vi "Untitled 25.vi"() -> ()   [LabVIEW 2019]
uses:
  examples/route_guide/route_guide_client/RPC Messages/routeguide_RouteSummary.ctl
  Generated_client/Generated_client.lvlib
  examples/route_guide/route_guide_client/route_guide_client.lvlib
panel:
  out "error out":errorcluster
  in  "error in":errorcluster
  in  "Longitude Loop":i32=4
  in  "Latitude Loop":i32=4
  in  "ms per iteration":u32=200
  out "Response Data":T1
  in  "Server Address":string="localhost:50051"
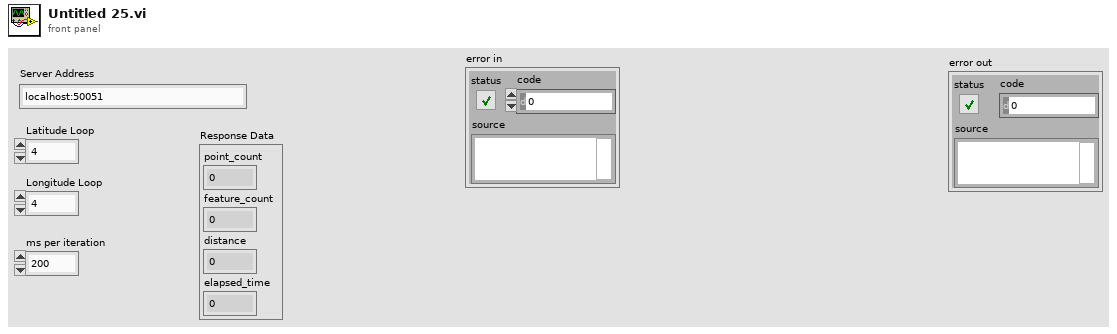
[diagram p1: front panel]
types:
  T1 = typedef "route_guide_client.lvlib/routeguide_RouteSummary.ctl" = cluster{"point_count":i32, "feature_count":i32, "distance":i32, "elapsed_time":i32}
  T2 = typedef "grpc-lvsupport-release.lvlib/grpcId.ctl" = u64
  T3 = typedef "Generated_client.lvlib/routeguide_RouteSummary.ctl" = cluster{"point_count":i32, "feature_count":i32, "distance":i32, "elapsed_time":i32}
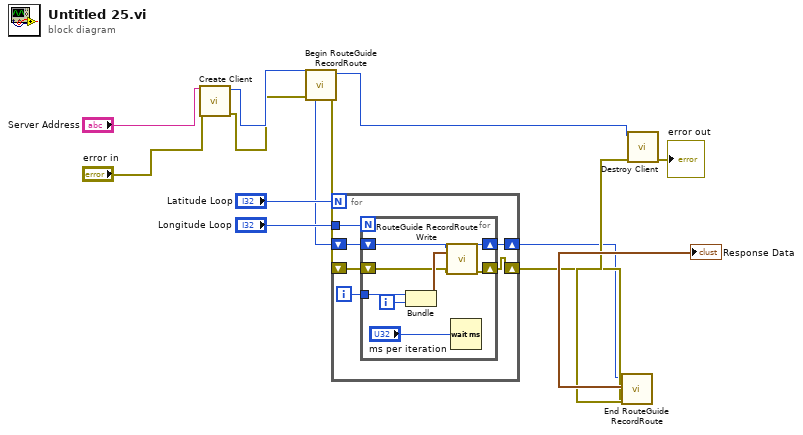
[diagram p0: block diagram]
diagram:
  n1 = call "Create Client.vi"("error in"="error in", "address"="Server Address") -> ("error out"=w5:errorcluster, "gRPC ID Out"=w9:T2)  [unwired: 8 in]
  n2 = call "Begin RouteGuide RecordRoute.vi"("error in"=w5, "gRPC ID"=w9) -> ("error out"=w6:errorcluster, "Call Id Out"=w7:T2, "gRPC ID out"=w8:T2)  [unwired: 7 in]
  n3 = for {
    N: "Latitude Loop" -> [_]
    shift-right: [w18] -> w1
    shift-left: w7 -> [w20]
    shift-right: [w15] -> w2
    shift-left: w6 -> [w19]
    tunnel: "Longitude Loop" -> [w16]
    i -> [w17]
    n4 = for {
      N: w16 -> [_]
      shift-right: [w22] -> w18
      shift-left: w20 -> [w25]
      shift-right: [w21] -> w15
      shift-left: w19 -> [w23]
      tunnel: w17 -> [w27]
      i -> [w28]
      n5 = Bundle(w27, w28) -> (w24:cluster{i32, i32})  [unwired: 1 in]
      n6 = call "RouteGuide RecordRoute Write.vi"("error in"=w23, "Request Data"=w24, "Call ID in"=w25) -> ("error out"=w21:errorcluster, "Call ID"=w22:T2)  [unwired: 6 in, 1 out]
      n7 = Wait (ms)(milliseconds to wait="ms per iteration") -> ()  [unwired: 1 out]
    }
  }
  n8 = call "End RouteGuide RecordRoute.vi"("error in"=w2, "Call ID in"=w1) -> ("error out"=w3:errorcluster, "Response Data"=→"Response Data":T3)  [unwired: 7 in, 1 out]
  n9 = call "Destroy Client.vi"("error in"=w3, "gRPC ID"=w8) -> ("error out"=→"error out":errorcluster)  [unwired: 9 in]
